vi "myRIO v1.0 Build MUX Configuration Encoder.vi"(11 "Channel":T4) -> (2 "Configuration Bitmask Array":bool[][](array[boolean]), 3 "Channel Reservation List":T1)   [LabVIEW 2021]
uses:
  <vilib>/myRIO/Common/Instrument Driver Framework/myRIO v1.0/Encoder/typedefs/Encoder Channels Enum.ctl
  <vilib>/myRIO/Common/Instrument Driver Framework/myRIO v1.0/Resource Manager/typedefs/myRIO v1.0 Channel Reservation List.ctl
  <vilib>/myRIO/Common/Instrument Driver Framework/myRIO v1.0/Resource Manager/typedefs/myRIO v1.0 Channel Reservation Info.ctl
  <vilib>/myRIO/Common/Instrument Driver Framework/myRIO v1.0/Resource Manager/typedefs/myRIO v1.0 Connector List.ctl
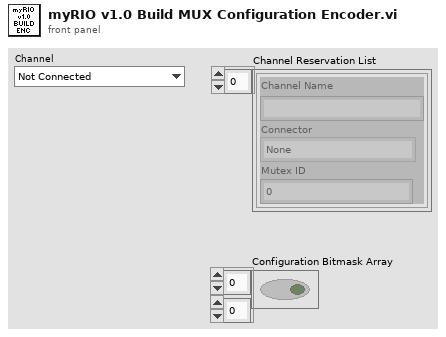
[diagram p1: front panel]
types:
  T1 = typedef "myRIO v1.0 Channel Reservation List.ctl" = T2[]
  T2 = typedef "myRIO v1.0 Channel Reservation Info.ctl" = cluster{"Channel Name":string, "Connector":T3, "Mutex ID":i32}
  T3 = typedef "myRIO v1.0 Connector List.ctl" = enum32{"None", "ConnectorA", "ConnectorB", "ConnectorC"}
  T4 = typedef "Encoder Channels Enum.ctl" = enum16{"Not Connected", "C/ENC0", "C/ENC1", "A/ENC", "A/ENC0", "A/ENC1", "A/ENC2", "A/ENC3", "A/ENC4", "A/ENC5", "A/ENC6", "A/ENC7", "A/ENC8", "A/ENC9", "B/ENC", "B/ENC0", "B/ENC1", "B/ENC2", "B/ENC3", "B/ENC4", "B/ENC5", "B/ENC6", "B/ENC7", "B/ENC8", "B/ENC9", "DIO/ENC0", "DIO/ENC1", "DIO/ENC2", "DIO/ENC3", "DIO/ENC4"}
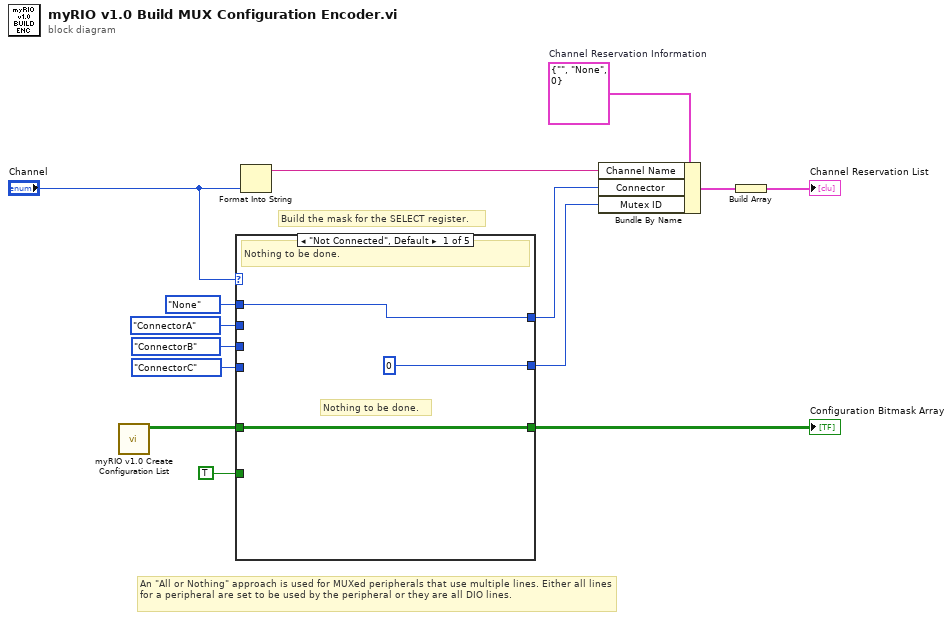
[diagram p0: block diagram]
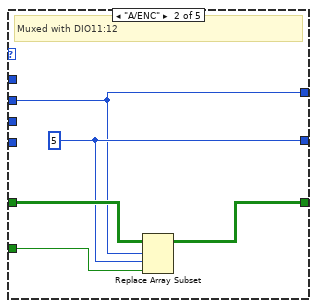
[diagram p2: hidden frame]
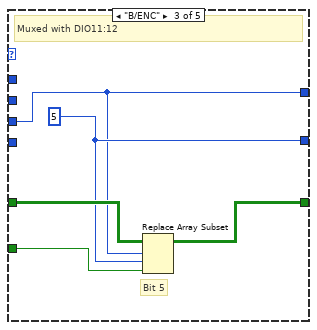
[diagram p3: hidden frame]
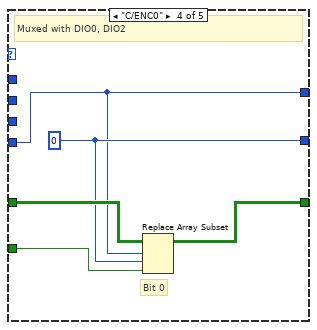
[diagram p4: hidden frame]
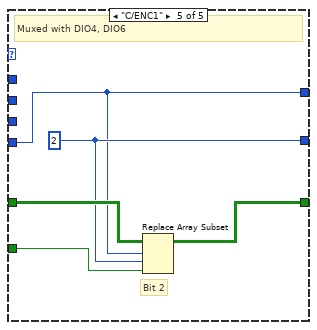
[diagram p5: hidden frame]
diagram:
  w6 = T2 {"Channel Name"="", "Connector"=enum."None", "Mutex ID"=0}  # Channel Reservation Information
  # "An \"All or Nothing\" approach is used for MUXed peripherals that use multiple lines. Either all lines for a peripheral are set to be used by the peripheral or they are all DIO lines."
  # "Build the mask for the SELECT register."
  n1 = call <vilib>:"myRIO v1.0 Create Configuration List.vi"() -> ("Bitmask Array"=w3:bool[][])  [unwired: 11 in]
  n2 = case shown="\"Not Connected\", Default" "Channel" {
    tunnel: w3 -> [w17 w22 w27 w32 w37]
    tunnel: [w17 w21 w26 w31 w36] -> w11
    tunnel: myRIO_v1.0_Connector_List."None" ("Connector List") -> [w16 _ _ _ _]
    tunnel: myRIO_v1.0_Connector_List."ConnectorA" ("Connector List") -> [_ w18 _ _ _]
    tunnel: TRUE ("new element/subarray") -> [_ w20 w25 w30 w35]
    tunnel: myRIO_v1.0_Connector_List."ConnectorB" ("Connector List") -> [_ _ w23 _ _]
    tunnel: myRIO_v1.0_Connector_List."ConnectorC" ("Connector List") -> [_ _ _ w28 w33]
    tunnel: [0 ("index") w19 w24 w29 w34] -> w1
    tunnel: [w16 w18 w23 w28 w33] -> w2
    frame "Not Connected", Default {
      # "Nothing to be done."
      # "Nothing to be done."
    }
    frame "A/ENC" {
      w19 = 5 ("index")
      # "Muxed with DIO11:12"
      n3 = Replace Array Subset(array=w22, new element=w20, index (row)=w18, index (col)=w19) -> (w21:bool[][])
    }
    frame "B/ENC" {
      w24 = 5 ("index")
      # "Bit 5"
      # "Muxed with DIO11:12"
      n4 = Replace Array Subset(array=w27, new element=w25, index (row)=w23, index (col)=w24) -> (w26:bool[][])
    }
    frame "C/ENC0" {
      w29 = 0 ("index")
      # "Bit 0"
      # "Muxed with DIO0, DIO2"
      n5 = Replace Array Subset(array=w32, new element=w30, index (row)=w28, index (col)=w29) -> (w31:bool[][])
    }
    frame "C/ENC1" {
      w34 = 2 ("index")
      # "Bit 2"
      # "Muxed with DIO4, DIO6"
      n6 = Replace Array Subset(array=w37, new element=w35, index (row)=w33, index (col)=w34) -> (w36:bool[][])
    }
  }
  "Configuration Bitmask Array" <- w11
  n7 = Format Into String("Channel") -> (resulting string=w5:string)  [unwired: 3 in, 1 out]
  n8 = Bundle By Name(cluster=w6, "Channel Name"=w5, "Connector"=w2, "Mutex ID"=w1) -> (w7:T2)
  n9 = Build Array(w7) -> (→"Channel Reservation List":T2[])
